vi "Copy block to VI.vi"(7 "Block path":path=path "C:/Projects/DMC/Autocomplete/Blocks/Other - Constructor.vi", 8 "error in (no error)":errorcluster, 9 "Object Label":string="Other - Constructor", 10 "position":T1, 11 "Target VI reference in":refnum<vi>) -> (0 "error out":errorcluster, 3 "Target VI reference out":refnum<vi>, 5 "GObject reference out":refnum<vi>)   [LabVIEW 2020]
uses:
  <vilib>/Utility/traverseref.llb/TRef TravTarget.ctl
  <vilib>/Utility/traverseref.llb/VI Scripting - Traverse.lvlib
  <vilib>/Utility/miscctls.llb/LVPositionTypeDef.ctl
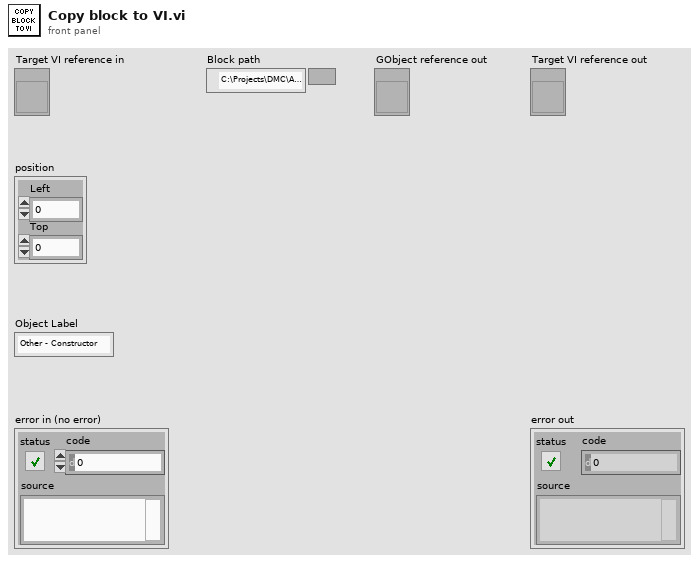
[diagram p1: front panel]
types:
  T1 = typedef "LVPositionTypeDef.ctl" = cluster{"Left":i32, "Top":i32}
  T2 = typedef "TRef TravTarget.ctl" = enum16{"FP", "BD", "Other"}
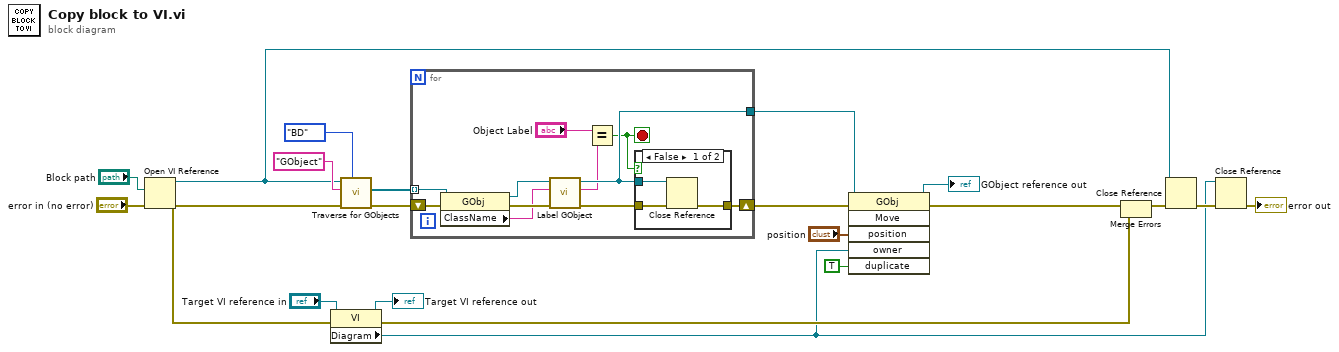
[diagram p0: block diagram]
diagram:
  n1 = Open VI Reference(vi path="Block path", error in (no error)="error in (no error)") -> (vi reference=w18:refnum<vi>, error out=w8:errorcluster)  [unwired: 4 in]
  n2 = property class="VI"(reference="Target VI reference in", error in=w8) -> (reference out=→"Target VI reference out":refnum<vi>, error out=w16:errorcluster, "Diagram"=w9:refnum<vi>)
  n3 = call <vilib>:"Traverse for GObjects.vi"("Traverse Target"=TRef_TravTarget."BD", "error in (no error)"=w8, "Class Name"="GObject", "VI Refnum"=w18) -> ("error out"=w15:errorcluster, "References"=w14:refnum<vi>[])  [unwired: 4 in, 2 out]
  n4 = for {
    shift-right: [w30] -> w12
    shift-left: w15 -> [w32]
    tunnel: w14 -> [w31] mode=indexing
    tunnel: [w25] -> w13
    stop <- w22 stop-if-true
    n5 = property class="GObj"(reference=w31, error in=w32) -> (reference out=w26:refnum<vi>, error out=w28:errorcluster, "ClassName"=w23:string)
    n6 = call "Label GObject.vi"("error in"=w28, "GObject ClassName"=w23, "GObject Reference In"=w26) -> ("error out"=w27:errorcluster, "Label"=w24:string, "GObject Reference out"=w25:refnum<vi>)  [unwired: 4 in, 2 out]
    n7 = Equal?(x="Object Label", y=w24) -> (x = y?=w22:bool)
    n8 = case shown="False" w22 {
      tunnel: w27 -> [w35 w36]
      tunnel: w25 -> [w34 _]
      tunnel: [w33 w36] -> w30
      frame False {
        n9 = Close Reference(reference=w34, error in (no error)=w35) -> (error out=w33:errorcluster)
      }
      frame True {
      }
    }
  }
  n10 = invoke class="GObj" method="Move"(reference=w13, error in=w12, "position"="position", "owner"=w9, "duplicate"=TRUE ("Duplicate? (F)")) -> (reference out=→"GObject reference out":refnum<vi>, error out=w11:errorcluster)  [unwired: 1 in, 4 out]
  n11 = Merge Errors(w11, w16) -> (w10:errorcluster)
  n12 = Close Reference(reference=w18, error in (no error)=w10) -> (error out=w17:errorcluster)
  n13 = Close Reference(reference=w9, error in (no error)=w17) -> (error out=→"error out":errorcluster)
